vi "monochromatorGetResponseINT.vi"(8 "error in":errorcluster, 10 "command":string, 11 "monochromator":refnum<k24>) -> (0 "error out":errorcluster, 2 "response":i32, 3 "reference out":refnum<k24>)   [LabVIEW 2009]
doc: "This VI accepts string command and returns response from the monochromator as INT\nBoth the command and monochromator vars are required\nIf connected error cluster contains error, command will not be sent and this VI will return -1 as response. \n\n<b>Warning:</b> It's unlikely, but possible that response value \"-1\" could be a valid response. Refere to monochromator programming manual for more information"
uses:
  C:/Users/anderson.chen/Desktop/Software Development/Cornerstone Series API (LV9)/Cornerstone DLL/Cornerstone.dll
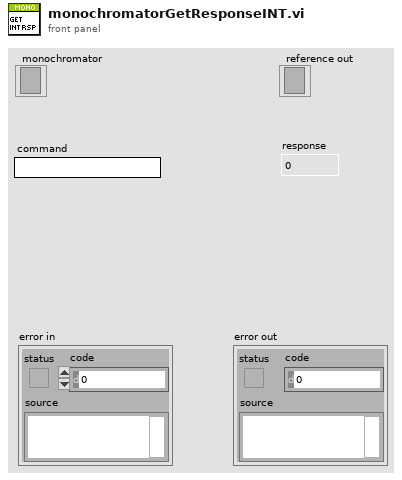
[diagram p1: front panel]
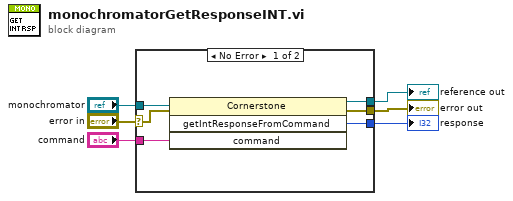
[diagram p0: block diagram]
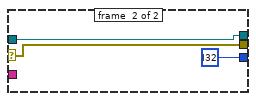
[diagram p2: hidden frame]
diagram:
  n1 = case shown="No Error" "error in" {
    selector: "error in" -> [w7 w15]
    tunnel: "monochromator" -> [w12 w14]
    tunnel: "command" -> [w11 _]
    tunnel: [w10 i32 ? ("getDoubleResponseFromCommand")] -> w4
    tunnel: [w9 w14] -> w3
    tunnel: [w8 w15] -> w2
    frame #0 {
      n2 = invoke class="Cornerstone" method="getIntResponseFromCommand"(reference=w12, error in=w7, "command"=w11) -> (reference out=w9:refnum<k24>, error out=w8:errorcluster, "getIntResponseFromCommand"=w10:i32)  [unwired: 1 in, 1 out]
    }
    frame #1 {
    }
  }
  "response" <- w4
  "reference out" <- w3
  "error out" <- w2
